vi "sub_psk_demod.vi"(8 "index map":i32[](array[numeric]), 9 "symbol map":cdb[](array[numeric]), 11 "symbol":cdb[](array[numeric])) -> (3 "bitstream":i16[](array[numeric]))   [LabVIEW 2014]
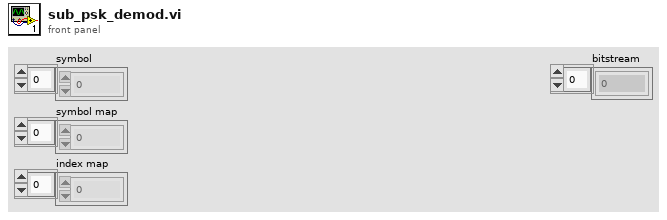
[diagram p1: front panel]
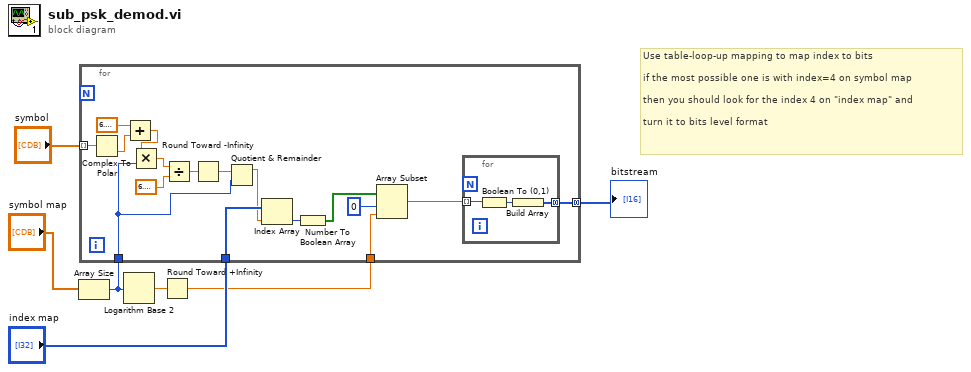
[diagram p0: block diagram]
diagram:
  # "Use table-loop-up mapping to map index to bits\n\nif the most possible one is with index=4 on symbol map\n\nthen you should look for the index 4 on \"index map\" and\n\nturn it to bits level format"
  n1 = Array Size(array="symbol map") -> (size(s)=w4:i32)
  n2 = Logarithm Base 2(1:w4) -> (0:w5:dbl)
  n3 = Round Toward +Infinity(x=w5) -> (ceil(x): smallest int >= x=w2:dbl)
  n4 = for {
    tunnel: "symbol" -> [w24] mode=indexing
    tunnel: w4 -> [w10]
    tunnel: "index map" -> [w21]
    tunnel: w2 -> [w17]
    tunnel: [w16] -> w1 mode=concatenating
    n5 = Complex To Polar(r * e^(i*theta)=w24) -> (theta=w13:dbl)  [unwired: 1 out]
    n6 = Add(x=6.283185307179586, y=w13) -> (x+y=w12:dbl)
    n7 = Multiply(x=w12, y=w10) -> (x*y=w22:dbl)
    n8 = Divide(x=w22, y=6.283185307179586) -> (x/y=w20:dbl)
    n9 = Round Toward -Infinity(1:w20) -> (0:w11:dbl)
    n10 = Quotient & Remainder(x=w11, y=w10) -> (x-y*floor(x/y)=w9:dbl)  [unwired: 1 out]
    n11 = Index Array(array=w21, index=w9) -> (element=w19:i32)
    n12 = Number To Boolean Array(number=w19) -> (Boolean array=w18:bool[])
    n13 = Array Subset(array=w18, index=0, length=w17) -> (w8:bool[])
    n14 = for {
      tunnel: w8 -> [w27] mode=indexing
      tunnel: [w25] -> w16 mode=concatenating
      n15 = Boolean To (0,1)(Boolean=w27) -> (0, 1=w26:i16)
      n16 = Build Array(w26) -> (w25:i16[])
    }
  }
  "bitstream" <- w1
